vi "Add Subordinate.vi"(8 "error in":errorcluster, 10 "Subordinate":T1, 11 "Manual UI in":refnum<class "Manual UI.lvclass">) -> (0 "error out":errorcluster, 3 "Manual UI out":refnum<class "Manual UI.lvclass">)   [LabVIEW 2019, in "Manual UI.lvlib" / "Manual UI.lvclass"]
uses:
  Project/Manual UI.lvclass
  builds/Engine/Actor Framework.lvlibp/1abvi3w/vi.lib/ActorFramework/Message Enqueuer/Message Enqueuer.lvclass
  Project/Manual UI.lvclass/Manual UI.ctl
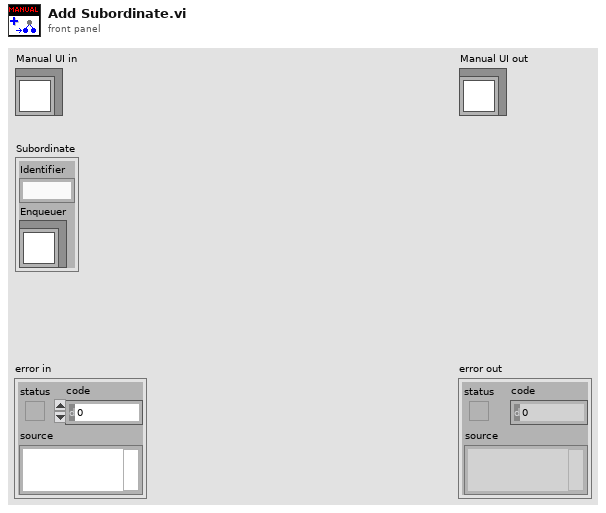
[diagram p1: front panel]
types:
  T1 = cluster{"Identifier":string, "Enqueuer":refnum<class "Message Enqueuer.lvclass">}
  T2 = cluster{"Identifier":string, "Enqueuer":refnum<class "Message Enqueuer.lvclass">}[]
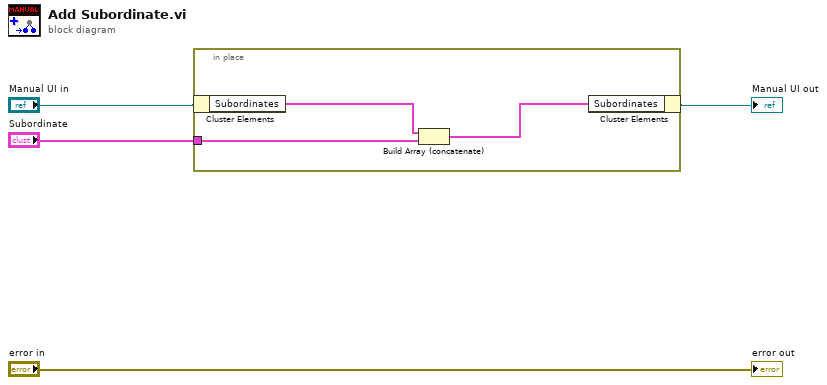
[diagram p0: block diagram]
diagram:
  n1 = in-place {
    in-place-border: "Subordinate" -> [w5]
    n2 = in-place-cluster #1("Manual UI in") -> ("Subordinates"=w7:T2)
    n3 = Build Array (concatenate)(w7, w5) -> (w6:T2)
    n4 = in-place-cluster #1("Subordinates"=w6) -> (→"Manual UI out":refnum<class "Manual UI.lvclass">)
  }
  "error out" <- "error in"
